vi "Disconnect.vi"(8 "error in":errorcluster, 11 "NCD in":refnum<class "ProXR.lvclass">) -> (0 "error out":errorcluster, 3 "NCD out":refnum<class "ProXR.lvclass">)   [LabVIEW 2019, in "ProXR.lvlib" / "ProXR.lvclass"]
uses:
  Library/ProXR.lvclass
  Library/ProXR.lvclass/ProXR.ctl
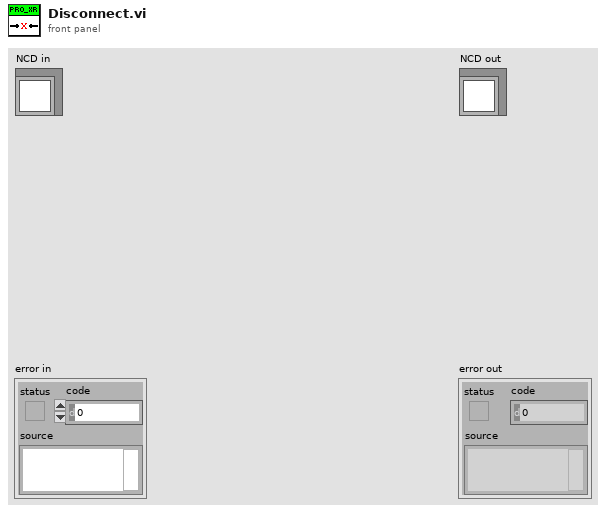
[diagram p1: front panel]
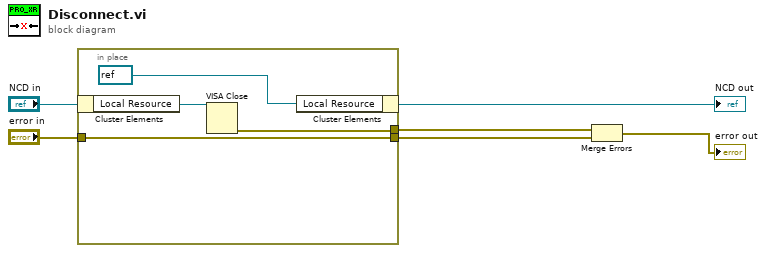
[diagram p0: block diagram]
diagram:
  n1 = in-place {
    in-place-border: [w8] -> w4
    in-place-border: [w7] -> w2
    in-place-border: "error in" -> [w7]
    n2 = in-place-cluster #1("NCD in") -> ("Local Resource"=w10:refnum<visa-resource-name>)
    n3 = VISA Close(VISA resource name=w10) -> (error out=w8:errorcluster)  [unwired: 1 in]
    n4 = in-place-cluster #1("Local Resource"=refnum<visa-resource-name> refnum) -> (→"NCD out":refnum<class "ProXR.lvclass">)
  }
  n5 = Merge Errors(w4, w2) -> (→"error out":errorcluster)
